vi "DecodeRegisterReply.vi"(2 "error in (no error)":errorcluster, 3 "Response":string="HTTP/1.0 200 OK\r\nServer: BaseHTTP/0.3 Python/2.7.1\r\nDate: Fri, 24 May 2013 07:09:25 GMT\r\nContent-type: text/xml\r\nContent-length: 296\r\n\r\n<?xml version='1.0'?>\n<methodResponse>\n<params>\n<param>\n<value><array><data>\n<value><int>1</int></value>\n<value><string>Unregistered [/labview] as provider of [/robot/head/command_head_nod]</string></value>\n<value><int>1</int></value>\n</data></array></value>\n</param>\n</params>\n</methodResponse>\n") -> (0 "error out":errorcluster, 1 "Reply":T1(array[cluster]))   [LabVIEW 2012]
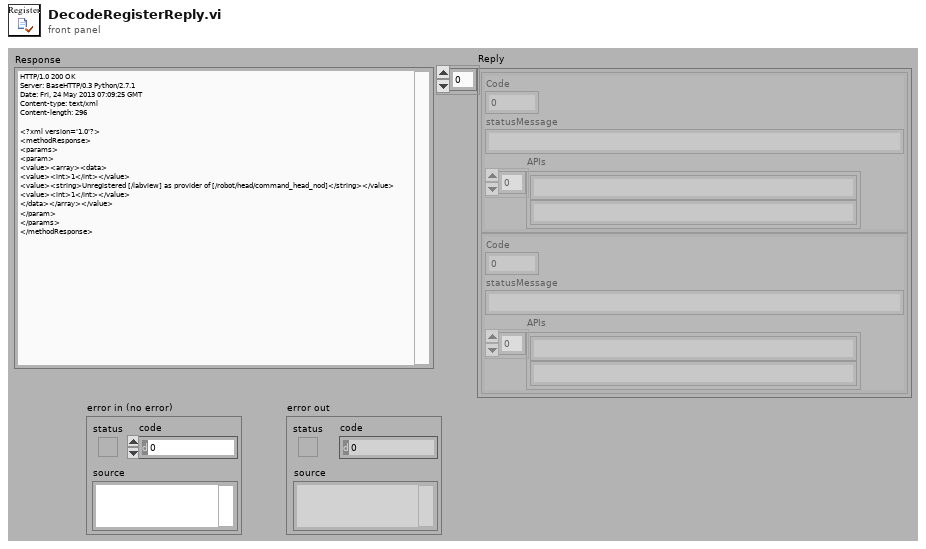
[diagram p1: front panel]
types:
  T1 = cluster{"Code":i8, "statusMessage":string, "APIs":string[]}[]
  T2 = cluster{"Code":i8, "statusMessage":string, "APIs":string[]}
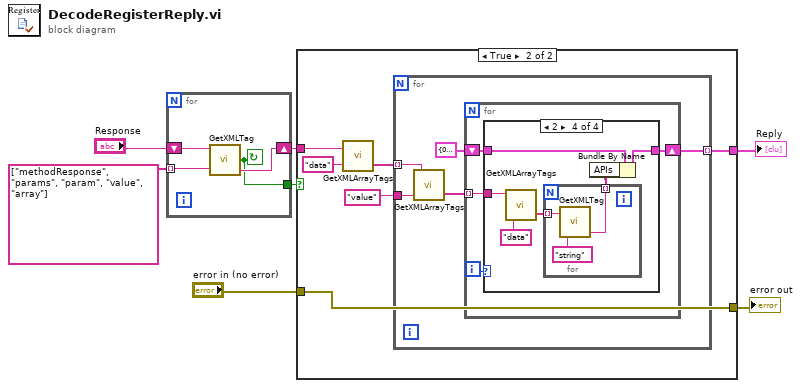
[diagram p0: block diagram]
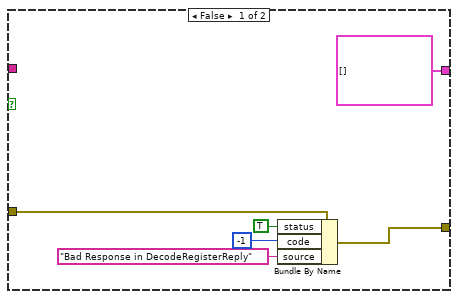
[diagram p2: hidden frame]
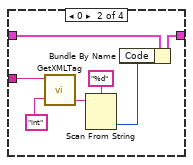
[diagram p4: hidden frame]
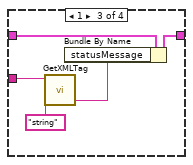
[diagram p5: hidden frame]
diagram:
  n1 = for {
    tunnel: string[] ["methodResponse", "params", "param", "value", "array"] -> [w11] mode=indexing
    shift-right: [w9] -> w5
    shift-left: "Response" -> [w10]
    tunnel: [w8] -> w3
    stop <- w8 continue-if-true
    n2 = call <userlib>:"GetXMLTag.vi"("Tag"=w11, "String"=w10) -> ("Value"=w9:string, "Exists?"=w8:bool)  [unwired: 1 out]
  }
  n3 = case shown="True" w3 {
    tunnel: w5 -> [_ w20]
    tunnel: [T1 [] w19] -> w4
    tunnel: "error in (no error)" -> [w16 w18]
    tunnel: [w15 w18] -> w1
    frame False {
      n4 = Bundle By Name(cluster=w16, "status"=TRUE, "code"=-1, "source"="Bad Response in DecodeRegisterReply") -> (w15:errorcluster)
    }
    frame True {
      n5 = call <userlib>:"GetXMLArrayTags.vi"("ArrayTag"="data", "String"=w20) -> ("Array"=w22:string[])  [unwired: 1 out]
      n6 = for {
        tunnel: w22 -> [w28] mode=indexing
        tunnel: "value" -> [w27]
        tunnel: [w24] -> w19 mode=indexing
        n7 = call <userlib>:"GetXMLArrayTags.vi"("ArrayTag"=w27, "String"=w28) -> ("Array"=w26:string[])  [unwired: 1 out]
        n8 = for {
          tunnel: w26 -> [w32] mode=indexing
          shift-right: [w29] -> w24
          shift-left: T2 {"Code"=0, "statusMessage"="", "APIs"=[]} ("Parameters") -> [w30]
          i -> [w31]
          n9 = case shown="2" w31 {
            tunnel: w32 -> [_ w39 w44 w49]
            tunnel: w30 -> [w33 w36 w43 w51]
            tunnel: [w33 w34 w42 w50] -> w29
            frame Default {
            }
            frame 0 {
              n10 = call <userlib>:"GetXMLTag.vi"("Tag"="int", "String"=w39) -> ("Value"=w38:string)  [unwired: 2 out]
              n11 = Scan From String(format string="%d", input string=w38) -> (output 1=w35:i32)  [unwired: 3 in, 3 out]
              n12 = Bundle By Name(cluster=w36, "Code"=w35) -> (w34:T2)
            }
            frame 1 {
              n13 = call <userlib>:"GetXMLTag.vi"("Tag"="string", "String"=w44) -> ("Value"=w41:string)  [unwired: 2 out]
              n14 = Bundle By Name(cluster=w43, "statusMessage"=w41) -> (w42:T2)
            }
            frame 2 {
              n15 = call <userlib>:"GetXMLArrayTags.vi"("ArrayTag"="data", "String"=w49) -> ("Array"=w47:string[])  [unwired: 1 out]
              n16 = for {
                tunnel: w47 -> [w54] mode=indexing
                tunnel: [w52] -> w46 mode=indexing
                n17 = call <userlib>:"GetXMLTag.vi"("Tag"="string", "String"=w54) -> ("Value"=w52:string)  [unwired: 2 out]
              }
              n18 = Bundle By Name(cluster=w51, "APIs"=w46) -> (w50:T2)
            }
          }
        }
      }
    }
  }
  "Reply" <- w4
  "error out" <- w1
